vi "System Testing Driver.vi"() -> ()   [LabVIEW 2009]
doc: "This VI will use the TLC modules to create a set of random Cues. The user specifies the number of Cues, and a TLC readable file will be created using the File Module."
uses:
  Modules/File/tlc_File_Command Control.ctl
  Modules/Cue/tlc_Cue_Information Command.ctl
panel:
  in  "Number of Cues":i32
  in  "Maximum Wait Time":dbl min=0.0 step=1.0
  in  "Maximum Fade Time":dbl=1.0 min=1.0 step=1.0
  in  "Maximum Follow Time":dbl min=0.0 step=1.0
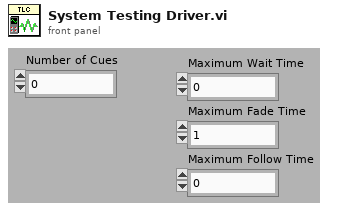
[diagram p1: front panel]
types:
  T1 = typedef "tlc_File_Command Control.ctl" = enum16{"Initialize", "Save Cues", "Load Cues", "Shutdown"}
  T2 = typedef "tlc_Cue_Information Command.ctl" = enum16{"Add Cue", "Get Cue Values", "Set Cue Values", "Get Number of Cues", "Initialize", "Get Empty Cue"}
  T3 = typedef "tlc_Cue_Information.ctl" = cluster{"Cue Name":string, "Wait Time (s)":u32, "Fade Time (s)":u32, "Follow Time (s)":u32, "Channels":T4[][]}
  T4 = typedef "channel.ctl" = cluster{"Intensity":dbl, " Color":u32, "Channel":i32}
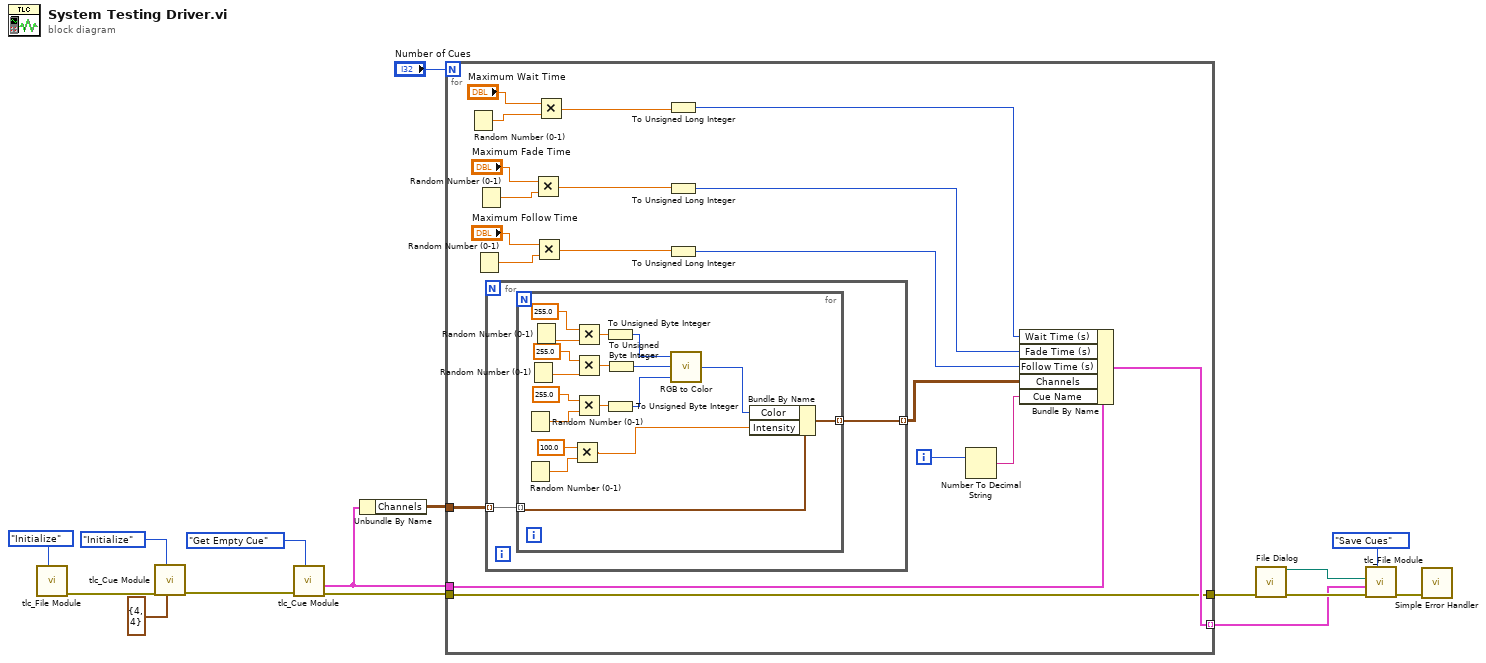
[diagram p0: block diagram]
diagram:
  n1 = call "tlc_File Module.vi"("Command"=tlc_File_Command_Control."Initialize") -> ("error out"=w14:errorcluster)  [unwired: 9 in, 1 out]
  n2 = call "tlc_Cue Module.vi"("Number of Channels"=cluster{"Rows":i32, "Columns":i32} {"Rows"=4, "Columns"=4}, "Command"=tlc_Cue_Information_Command."Initialize", "error in (no error)"=w14) -> ("error out"=w15:errorcluster)  [unwired: 5 in, 2 out]
  n3 = call "tlc_Cue Module.vi"("Command"=tlc_Cue_Information_Command."Get Empty Cue", "error in (no error)"=w15) -> ("error out"=w16:errorcluster, "Cue Output"=w9:T3)  [unwired: 6 in, 1 out]
  n4 = Unbundle By Name(w9) -> ("Channels"=w8:T4[][])
  n5 = for {
    N: "Number of Cues" -> [_]
    tunnel: w16 -> [w20]
    tunnel: w9 -> [w26]
    tunnel: [w21] -> w1 mode=indexing
    tunnel: [w20] -> w4
    tunnel: w8 -> [w19]
    i -> [w18]
    n6 = Random Number (0-1)() -> (number: 0 to 1=w34:dbl)
    n7 = Random Number (0-1)() -> (number: 0 to 1=w30:dbl)
    n8 = Random Number (0-1)() -> (number: 0 to 1=w32:dbl)
    n9 = for {
      tunnel: [w37] -> w25 mode=indexing
      tunnel: w19 -> [w36] mode=indexing
      n10 = for {
        tunnel: [w39] -> w37 mode=indexing
        tunnel: w36 -> [w38] mode=indexing
        n11 = Random Number (0-1)() -> (number: 0 to 1=w54:dbl)
        n12 = Random Number (0-1)() -> (number: 0 to 1=w43:dbl)
        n13 = Random Number (0-1)() -> (number: 0 to 1=w55:dbl)
        n14 = Random Number (0-1)() -> (number: 0 to 1=w53:dbl)
        n15 = Multiply(x=100.0, y=w43) -> (x*y=w41:dbl)
        n16 = Multiply(x=255.0, y=w53) -> (x*y=w49:dbl)
        n17 = Multiply(x=255.0, y=w55) -> (x*y=w47:dbl)
        n18 = Multiply(x=255.0, y=w54) -> (x*y=w44:dbl)
        n19 = To Unsigned Byte Integer(number=w49) -> (unsigned 8bit integer=w48:u8)
        n20 = To Unsigned Byte Integer(number=w44) -> (unsigned 8bit integer=w45:u8)
        n21 = To Unsigned Byte Integer(number=w47) -> (unsigned 8bit integer=w46:u8)
        n22 = call <vilib>:"RGB to Color.vi"("B"=w45, "G"=w46, "R"=w48) -> ("Color"=w40:u32)
        n23 = Bundle By Name(cluster=w38, "Color"=w40, "Intensity"=w41) -> (w39:T4)
      }
    }
    n24 = Multiply(x="Maximum Fade Time", y=w32) -> (x*y=w28:dbl)
    n25 = Multiply(x="Maximum Follow Time", y=w30) -> (x*y=w29:dbl)
    n26 = Multiply(x="Maximum Wait Time", y=w34) -> (x*y=w27:dbl)
    n27 = To Unsigned Long Integer(number=w27) -> (unsigned 32bit integer=w22:u32)
    n28 = To Unsigned Long Integer(number=w28) -> (unsigned 32bit integer=w23:u32)
    n29 = To Unsigned Long Integer(number=w29) -> (unsigned 32bit integer=w24:u32)
    n30 = Number To Decimal String(number=w18) -> (decimal integer string=w17:string)  [unwired: 1 in]
    n31 = Bundle By Name(cluster=w26, "Wait Time (s)"=w22, "Fade Time (s)"=w23, "Follow Time (s)"=w24, "Channels"=w25, "Cue Name"=w17) -> (w21:T3)
  }
  n32 = call "File Dialog"("error in"=w4) -> ("selected path"=w2:path, "error out"=w3:errorcluster)  [unwired: 11 in, 2 out]
  n33 = call "tlc_File Module.vi"("Command"=tlc_File_Command_Control."Save Cues", "error in (no error)"=w3, "Cue Array Input"=w1, "Path"=w2) -> ("error out"=w6:errorcluster)  [unwired: 6 in, 1 out]
  n34 = call <vilib>:"Simple Error Handler.vi"("error in (no error)"=w6) -> ()  [unwired: 4 in, 5 out]
